vi "Calc Pitch.vi"(10 "Position":dbl) -> (2 "Pitch":dbl)   [LabVIEW 2014]
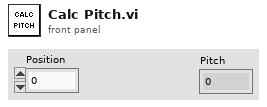
[diagram p1: front panel]
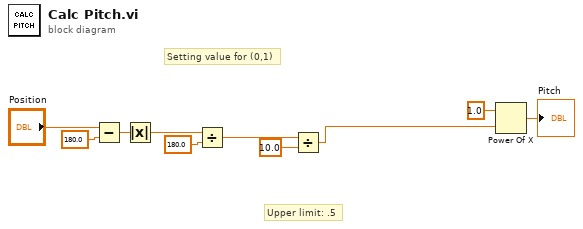
[diagram p0: block diagram]
diagram:
  # "Upper limit: .5"
  # "Setting value for (0,1)"
  n1 = Subtract(x="Position", y=180.0) -> (x-y=w8:dbl)
  n2 = Absolute Value(x=w8) -> (abs(x)=w7:dbl)
  n3 = Divide(x=w7, y=180.0) -> (x/y=w3:dbl)
  n4 = Divide(x=w3, y=10.0) -> (x/y=w2:dbl)
  n5 = Power Of X(1:w2, 2:1.0 ("y")) -> (0:→"Pitch":dbl)
